vi "GetXL_AllCellValues.vi"(8 "error in (no error)":errorcluster, 11 "Refnum Cluster Out in":T1) -> (0 "error out":errorcluster, 2 "data":string[][](array[string]), 3 "Refnum Cluster Out out":T1)   [LabVIEW 2017, in "excel_configuration.lvlib"]
uses:
  excel_configuration.lvlib
  GetXL_CellValues_2D_String.vi
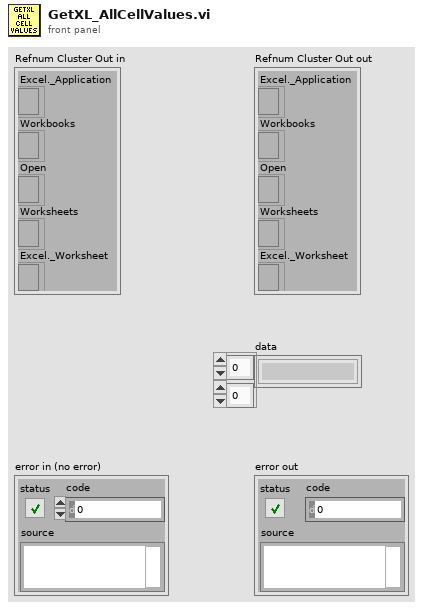
[diagram p1: front panel]
types:
  T1 = cluster{"Excel._Application":refnum<k7>, "Workbooks":refnum<k7>, "Open":refnum<k7>, "Worksheets":refnum<k7>, "Excel._Worksheet":refnum<k7>}
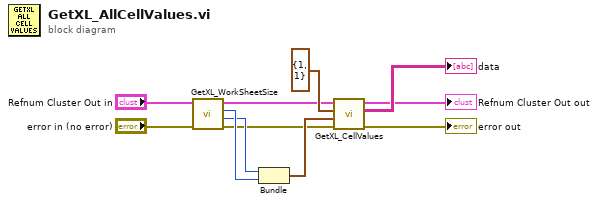
[diagram p0: block diagram]
diagram:
  n1 = call "GetXL_WorkSheetSize.vi"("error in (no error)"="error in (no error)", "Refnum Cluster in"="Refnum Cluster Out in") -> ("error out"=w5:errorcluster, "# Columns"=w8:i32, "# Rows"=w9:i32, "Refnum Cluster Out"=w3:T1)  [unwired: 6 in]
  n2 = Bundle("# Columns"=w8, "# Rows"=w9) -> (w7:cluster{"# Columns":i32, "# Rows":i32})  [unwired: 1 in]
  n3 = call-poly "GetXL_CellValues.vi"("error in"=w5, "End"=w7, "Start"=cluster{"Column":i32, "Row":i32} {"Column"=1, "Row"=1}, "Refnum Cluster In"=w3) -> ("error out"=→"error out":errorcluster, "data"=→"data":string[][], "Refnum Cluster Out"=→"Refnum Cluster Out out":T1)  [unwired: 5 in]
